vi "Queue_Status_GUI (SubVI).vi"(8 "error in (no error)":errorcluster, 11 "Queue in":refnum<queue>) -> ()   [LabVIEW 2017]
uses:
  Global_SNK3_HF.vi
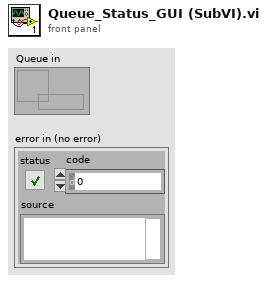
[diagram p1: front panel]
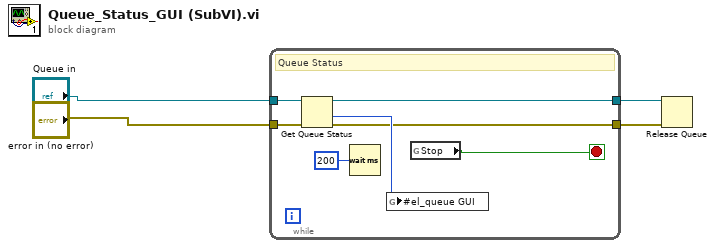
[diagram p0: block diagram]
diagram:
  n1 = while {
    tunnel: "Queue in" -> [w11]
    tunnel: [w5] -> w2
    tunnel: "error in (no error)" -> [w10]
    tunnel: [w9] -> w1
    stop <- w6 stop-if-true
    # "Queue Status"
    n2 = Get Queue Status(queue=w11, error in (no error)=w10) -> (queue out=w9:refnum<queue>, # pending insert=w7:i32, error out=w5:errorcluster)  [unwired: 6 out]
    n3 = Wait (ms)(milliseconds to wait=u32 200) -> ()  [unwired: 1 out]
    n4 = global write "Global_SNK3_HF.vi" "#el_queue GUI"(w7) -> ()
    n5 = global read "Global_SNK3_HF.vi" "Stop"() -> (w6:bool)
  }
  n6 = Release Queue(queue=w1, error in (no error)=w2) -> ()  [unwired: 4 out]
